vi "Parse Data Out.vi"(0 "Raw Data In":string, 11 "Error In":errorcluster) -> (4 "Data Out":T1 {"CRC" format="%04x"; "Length" format="%02x"; "Command" format="%02x"; "Destination" format="%02x"; "Source" format="%02x"}, 15 "Error Out":errorcluster)   [LabVIEW 2014, in "GEA2_Toolkit.lvlib"]
uses:
  library/GEA2_Toolkit.lvlib
  type defs/Data Out.ctl
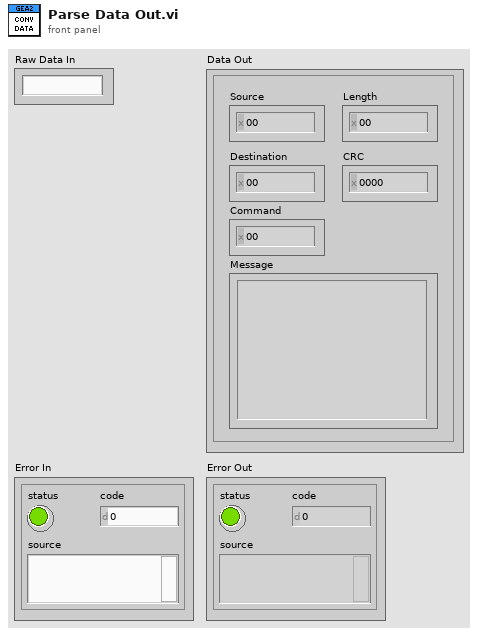
[diagram p1: front panel]
types:
  T1 = typedef "GEA2_Toolkit.lvlib/Data Out.ctl" = cluster{"Source":u8, "Destination":u8, "Command":u8, "Length":u8, "CRC":u16, "Message":string}
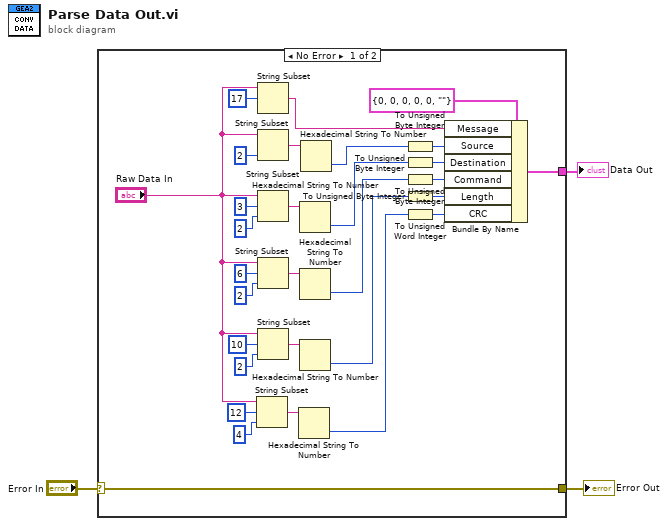
[diagram p0: block diagram]
diagram:
  n1 = case shown="No Error" "Error In" {
    selector: "Error In" -> [w26 w34]
    tunnel: [w26 w34] -> w2
    tunnel: [w15 _] -> w1
    frame No Error {
      n2 = String Subset(string="Raw Data In", offset (0)=12, length (rest)=4 ("length (rest)")) -> (substring=w6:string)
      n3 = String Subset(string="Raw Data In", offset (0)=17) -> (substring=w27:string)  [unwired: 1 in]
      n4 = String Subset(string="Raw Data In", length (rest)=2 ("length (rest)")) -> (substring=w23:string)  [unwired: 1 in]
      n5 = String Subset(string="Raw Data In", offset (0)=3, length (rest)=2 ("length (rest)")) -> (substring=w25:string)
      n6 = String Subset(string="Raw Data In", offset (0)=6, length (rest)=2 ("length (rest)")) -> (substring=w24:string)
      n7 = String Subset(string="Raw Data In", offset (0)=10, length (rest)=2 ("length (rest)")) -> (substring=w14:string)
      n8 = Hexadecimal String To Number(string=w6) -> (number=w4:u32)  [unwired: 2 in, 1 out]
      n9 = Hexadecimal String To Number(string=w25) -> (number=w18:u32)  [unwired: 2 in, 1 out]
      n10 = Hexadecimal String To Number(string=w24) -> (number=w17:u32)  [unwired: 2 in, 1 out]
      n11 = Hexadecimal String To Number(string=w14) -> (number=w10:u32)  [unwired: 2 in, 1 out]
      n12 = Hexadecimal String To Number(string=w23) -> (number=w22:u32)  [unwired: 2 in, 1 out]
      n13 = To Unsigned Byte Integer(number=w22) -> (unsigned 8bit integer=w21:u8)
      n14 = To Unsigned Byte Integer(number=w18) -> (unsigned 8bit integer=w20:u8)
      n15 = To Unsigned Byte Integer(number=w17) -> (unsigned 8bit integer=w19:u8)
      n16 = To Unsigned Byte Integer(number=w10) -> (unsigned 8bit integer=w11:u8)
      n17 = To Unsigned Word Integer(number=w4) -> (unsigned 16bit integer=w9:u16)
      n18 = Bundle By Name(cluster=T1 {"Source"=0, "Destination"=0, "Command"=0, "Length"=0, "CRC"=0, "Message"=""} ("Data Out"), "Message"=w27, "Source"=w21, "Destination"=w20, "Command"=w19, "Length"=w11, "CRC"=w9) -> (w15:T1)
    }
    frame Error {
    }
  }
  "Error Out" <- w2
  "Data Out" <- w1
